vi "Part 1.vi"(11 "Input":string="^^<<v<<v><v^^<><>^^<v<v^>>^^^><^>v^>v><><><<vv^^<^>^^<v^>v>v^v>>>^<>v<^<v^><^>>>>><<v>>^>>^>v^>><<^>v>v<>^v^v^vvv><>^^>v><v<><>^><^^<vv^v<v>^v>>^v^>v><>v^<vv>^><<v^>vv^<<>v>>><<<>>^<vv<^<>^^vv>>>^><<<<vv^v^>>><><^>v<>^>v<v^v<^vv><^v^><<<<>^<>v>^v>v<v<v<<>v<^<<<v>>>>>^^v>vv^^<>^<>^^^^<^^^v<v^^>v<^^v^^>v>^v^^^^>><<v<>v<>^v^<v<>><>^^><<^^<^^>vv<>v^<^v<vv<<<>^>^^>^<>v^^vv<>>v><<<>vvv<>v<>><^<^v<>^vv>^^v<v<v><^<>>vv<^>>^>>vv^v<vv^vv<^<<>>^v^<>^>>>>vv>^^>v>vv>v><^vv^<<v>^<<^^<v<v>vv<v^^<>^^v>^>>v><^<<vv<<v^vv^^^v>>v<<v^><vv^><vv<^vv<<vv^v<<^v<^^v>><<v^>>^^<>v>><<v<>>^^<v>>^^>>vvv^><<<<<^<^vv<^<><v<<>^^^<<<^>^^^<v<<vv>vv<>^<>v<^v>^<<<v<v<v>>^v<>>v<<^<<v<<>^<<<><><>^>>>>^>v^v<<v<v<<>>vv<^vvv^^^^<vv>vv>^v^^v^<v^v><^vv<^vv>v<^>vv<>>^>^><vv<><^>v>^v>vvv<>^>^v<><>vv>><^v^<><><v>>v^v^><^<^>vv>v<^>vvv>v<<<<<^<v<<vv<^^^<<>>^v<vv<^<>v>^<v<>><><>^<<v>v^>^<vv>><><>>^>^>><^<v>^^>^^>^^v^^<^v^^>v^^>>><<><v<v<<v^vv<><><>^<v>^<<^^v^>v>><>^^^><^vvv<^^^^^v><<><v<^^v><><>>^>vv<vvvv<<>>><v<^^^^v<<^><v>^vv<v^^v^vv<^^>^^<v>><<v^>v<^^>^<^<v<^^v>^<<v>^>>>^v<>v<^^^>vvv^v<<^><>>><vvv^<^^^<^>>v>>><v>^^vvv^vvv<^^^^v^v^<vv^<v>^<<^>v^v^<<><>><^v><v<><<>><<<>^v>v<>^<v^v>^vv>>^<>v^^<<v><^v>>v<>>^v^^>><^>v^<^v^^>><>v^>^v^v<<<v^<v^^v<^>v<><>vv>>>>^>v<>v<<<>^^>vv^v<><v^<>^<<<<>>^^>^v<v^v<<><>^v<>>^v^<<^<^>>>^vv<><v<^^<>v^>>v<^^v<v>>>^>><<><<<>><vv<v>>^v>><^<v><vv>^vv<v<>>><>v^><>vv<^^v^^^v<>><^vvv<<^<>v>>>v>><v><>>><>><v^><v^v<v>^v>v<v>>^^<^>^>v><>vv>^v><<>>>>>>>^<<^vv^^vvvv<^^><<<v<<>vvv<>^><<v<v^v^<<v>v<>>^<vv^<v<v>^<<^^vv>v>^<vv<<>v<v^<>v>>^v^^vvvv>^^>>v^v^^><<^>v>>^^>^<^^<>v<v>vv^vv>v<v>>^v<><^vv^<vv<v^^^v<^v^>>^v>>>^^<^<^>^v^>^>>>^v>^>^^^>>^<>v^^<>^v<<^^>^^<vv<>v<^v^>><^v^>^<>>^vv^vv^>v^<vvvvvv^>><^^<^v<^<v^<<^^<<v^<^>><>v><^v^v^^^v>v^<>^<<v<^^vvv<v>^^>^v^^<><vv^v^>v^<<>>vv<>>>>v>v<>^>>>v<>^^><v<v^^^<>^<^><>^><<v>><>^<<>>><<^<vvv<^><v>>^vv^v>><v<>vv^<<^^<<><v><<^<v<vv<<^v^vv>v^>>>v<<<<v<<>v>^vv<^v><v<v>v<^>^^vv>v><v>><<v<<v^v>>><>^<>><><<^<<^v^v<<v>v>v<v<^^>vv<^v^^^<v^<<<v<>v^><^v>^<^<v>>^<<<v>>v^<><>>^v<>vvv<vvvvv<^^><^>><^^>^>^v^vv<^><<^v>><^^v>^v<>^>vvvv><^>^<<v^^vv<v^^<><>v>^>>^<^<<<^v^^^>^>>^>><><<^>v^^<v>>v<<<<vvv<vvvv^<^<v^^<>^>vvv^<vv^v^v>^<<><v><^v^v^^^>^^>^vv<>v>>v^>vv^vv>v<^v^^>>^v^v<>>^^><<v<<>><>>>^>^<>^^v^^><^<>><<^<vv^^^^^>>vv^<v^<^>>>>v<<><<^>vv>vvv>^<><>>>>vv><<v^v<^^^<<^^^vv^<v<><><<<<>><<v^<>v>v^><>v^v^^><>v>v>^^v<^v<>>^^^^^<v>><v^>^^<v>><v^^>v<^<^>>>^><^^>><<>>^><>^^^>v^^^>^^v^<>^^><^>>><><^>>v<v^>v<^><v<v^<>v<^v>v^<^vv^^><<<><><^v^<v<^^>v>v^>>^^vv^<v>^v>^<^v<>^>^><^<v>^v><^<^<>v^^>^><>>><<v><<><>v<<^v^^<^><>^<><><v>v<^^<v<v>>^^<<>>^<v>><^><^<^>^^v<>v>>><><<>^>v><><<<<v^^^^v<>>^^^v>><<^v>^>>><vv^>>^vv<^<>>^<^^<^v>v<v<<<<<>^<<^<<<<<^<^>>^><<>><>v^v>^<^>v^<><vvv^>^v^v^v><^<v<>vv<<^<>^^^<>^v>^<v^^<v^v>v<>>^>v<<>v<>v^v>v<<<>>v>vv>>v<<>v<>v<^>^>^<v>>v>^>^^^<vv>v<<>>><v>^vvv^^>^^<^vv^^^^>v>^v^>v^^v^>>^v>^vv>^^v^<<<<>^<><^<^<<^^>v^^^v<>>vvv<v>>vv><v<v>^<^v>>^v<vv^<<v<vv><^^v^v>v<>^v<<<^^v^^^<^v>v^v^v>><vvv<<>v<>^v>vv^v>vv<<^v<v>^v>v>><^v<v<>v>>>><<<><vv><>^v^<^vvv>v<>><^v>^>><v>vv<><><>v><>>><^>vv>>^<>v^>>^><<<^><<>^v^>>><><>vv>^<>^>^v^^><^>>><<>v^<^vv>^<^vv>><v<>vv<v><><<^><>v<^^<^>vv^^^^vv<<v><>vv<><v>v<>>>>^><v><>^<><>v<>><<>^^vvv>^^^<><>>vvv^v>><>vv<vv>^^^v^<<>^^v<><<^^v<>^^>^<^^v>>v^v^^>>v>>>^<<^<>^>^^v>>>><vv<<>^v<<vv><<^^vv><^>vv<>>v<v>v^>v>>v^<vv<<<v><v^>vvv^^>vv^<<v>v^>>v^<>>><><<^^<^v>^>>>v>v>^v<>vv><vv<vvv<<v>v>^v<<<>><<><><>v^>>>v^>v^>>vv^^<v>^<>>><^>v^<>^^><v>v<><<<><v^v<<<v<v^>v^v>^>v<^<>v>v^^>>v>vv^v<>>^^^^<>v^>>>>>>>><v<^<<vvv<^v^>^v<^<<>>><<<^<<^>^>v^<>^<<<>v>><^vv^>^>^>>>^<vv><v^^^<v^<v<><v^vvv<>v<vvv^vv<<<v^<^<^vvvv^<<vv<^v><<>^>^<v^v^<^>v^><>>v^>v^>^>>v<>vv^v<<>^^>>vv<>vv>>^v<^vv>^v>v<v^vvv^<<^><>v^<><vv><>v^^><<<><>^>^v^<>><vv<^>v^v>v<>><v<<^>^<vv<^v>^<<v><^<^^vv^<>><v^>^vv^<>>^^^^v>v><^^^v^<<<>^<^<<>><>>v<<^v^>><><v^>>^vv^v>vv>>>>>>^^<<>v^>v^v>^^>>><vv^^^v>^v>>^^^<>><>v^<<<v<vv^^<v^<<<>v>v^^^<vv<>>^v>^v<^<<><>vv>^^^<^^vv<v<<vv>^^>vv>v<<^>^vv><^><v>^^^^v<<vv>v^<<^^>>^^vvvv^v^>vv>>v^<v>vvv<>>^><>>v^^>>^<>>vvvv^>><v^v<^^<^vv>>v<<^<<^><v^^><v^>v^>><<<v>v>v^>^v<v^vv<^^^v<^<vvvvv<<vvv>><>v<v<v<<^v<><<>vv>><v>><^>>^^v>^>><>vv^><<>>vv<<<^<^^>^<<^>>>><v<^v<<<>>v>vv<^>^v><>>v<v^v<>v^vvvv>v^>>v><<^<v>^^v>>vv^^>v>^v>^v^^>^<^vv<v<<^>vv<<^>>^<<^^>>^<^>v^><^vv>^^v><v^>>><>v^v>^v<^><<<>vv><v>v<><>>v^<>^^>^<>^<<^>>vv^><^<v<^^vvv>>v^>>v^>v>vv><>>v<^>><<<v<<vv><v<v<v>v<v>vv^vvv^vv^>^>v><vv<v^^<>>>>vv^>^<>v<^>^<^v>vv<^<<>>^<^<vv><^^<>^<<v^v^>v<<><v>v>><^v<<^vvv>v>v<<^^<^^>v<vv<v<v^v>^^^>^>vv<v<<^^v^<v<^>^^^vv>v<>>>vv>><><^><><<<vvv<<^^v^<v^<<^>>vv>vv^v^>>><v><<v^v>>v>>vv>^^vvv^>^^>^>^>^v<<^vv^>vvv^^vv><^>^v^>^><>v<^^vv<v><v^<><^<>><v>^^v^v>v^vv<>><^v>^<^v>^<>^v>>>><<vv^^^vv^>>><vv^v>>v><^v^vv><<^v<<>^^<v><^v>vvv<><^^><<^v><>^<^v<^^<^vvvv^^>>>>vv>v>>>v<v^><<<<v>>v^><v>>vv^v<vv<>vv<>vvv>>>><>>><>^v<v^v><vvv<<v^^v^v<>>><>>^vv<<v<><<vv<v^>^^vv><^v^v<v^vvv^v>v^^^vv>^><^vvv<<>^vvv^<v<v^v>>>>^<<<><<<<<^v<^^>>>>^>^<v^^^v<vvv<vv^<>v<<<^<^>>v^<v><<><<^^vvv^>v<>>^^>v>^v>>v<v><v>>>>^<^<^>v^v<vv<>^>><>^<<^vvv^^<>^<vvv<>v^>^^<<^>^vv><vvv>>v^v^>v><v>^<^^<>^>^>>>^^vvv^<<>v^<<>><>v<^<^>v^>^vv><v<^<<<^v>^>>^<^v^<<<<^v^><v^v>v^><<v<><<v^<<^<<v<<v><v><><^^^^>v>^^<v>>v<vvv<<<>><>>^><<><^<>>^^>vv<^><^v^><vvv>>>vvv<<vv^<^^^<^>^<>>^>>^v^<^^v>^<v<<>^^v<^vv^><vvv>>^v><<^<v^<><><>>^>vv<<>^^^v^^<v<>><>>vv>v^>vvv^^v<vv<^<^>>^>>^>>v^<<<v^>v^<^v^vv^><^<^v<<v<<>v>^v^<<<v^vv<v<<>^^<v>>>^<v<^>^^v<v>>>><vv<^^<<>><<v<v>^^v^>>^^>>^v^<^v>v^v^v^v^>v^vv<><>^^<>^><^^^<<<^<v>v<<>^<^^^^^v^<^<<^^>^vv<>v^>><>>^>v>v<>^>v<v^>>><>^<><v>>>^>^>>v^><v<>v><^vv^>v<<v>v<><<vv<<v>^><^<v^>v<<v^v<<><v><>v<v><>^^<v<>><<>v>vv<<v>^v<v>vv><><>vv^<<>^>^<^>>>^v>v<^v^^^vv<>>>^<<^>>><<^^v^>v^<^v>vvv>v^^vv>^^>>v<>^<<>^<><^^v^>><>^>v>>^^^<<^^v<>^^>^<>^>><^>^vvv><^>^<^>^>>vv<^>>^v>>^<>>^^>>>v^<v>>v<<v<^>>v^^vv>v><^v^^><vv^v<^>v<<>v^^<><>^>vvv><^^^>^v^>v>>^vvv<^vv>^^>^>>v<>><<^v<<v^>^><>vv^<<^^vv><v>>^<^><^<v>^v<v>^<<>^v^^>v^>>^^^<^vv>v^>>>vv<<>v>>>^>v^^<v^v^^v^>>v<v<<v>^<<>>vv<<^v>v<<vv<<^<^v<^<><^^>v>>v>v^>><vv<^v<^>^>>v>^><<^<<>^v<v>>><^^<^<<<v^^>^>vv<<>^<>^<v^<<^v>vv>^^^v<^v><v<<<<<vv>vv>^^^^>v>v><<^<<<^vv><^<<<><v>><v^v>v<<v^^<v^>v>^v^v^<^<^vv>vvv<^^v<>v<<<<>v<v^<vvv^^^<<^<^<<>^<<><<<>v<^>^^v<^^v^>vv>vvv>v><v^^<<>>^><^>>v<<vv>v<<^^^v<<^v^^><><<<><<>v>^<<>v<<<^v>><v^v<^v<v^vv>v>><<^<><^v^^v<v>^>^>vvvv<<><<>>^<vv>^^><v<>v>v<v^^>^><>>><^><<><<<^<>v^><vv^^^^>>^v^>v^<>>v>^^><^<^v^<v^>>v>^vvv<>>v<v^v><>^vvvv<v^<<v^<<^^vv>><<<<<<v><<<v<v^v^^<v^^<>v<<<<^v<<><<v^<^><v<vv<v^v^<v^^vv<v^v<<<>^<<>vv<v<^>^<<><vv<<vv<v<^<^<>><^^<<>>>vv>>>>>>^v<v<>>v^v^^<v^<<<<>><<^v^^^<>^<vv>>>><>v^v^vvv^>>v>><v^v<<<^v>>^^<<^^vv><<<^^^<<<v><^^>>>>vvv^v<^>^^>v<^<><vv<v<>v>>>^vv<<^<v>^v^>^>^v>v>v^v^>v<<v>><>><v^^<<^>>>><<^v^<>^v<vv><>vvv^>v>v<v<v^>^<><><>^>>><v<<<v^vv><>^>^^<<v^>>v^^>^<v>><>><>v^v^^v>>>>vv>>^v<<^v^<>^>v^^>^^<<vvvvvvv>^<v^<<^<<>><<<^^^v^^^^v<^<>v<^^<>vv^^v^<>^<<^>>v>v<<<^^^^vvv^<^<><>v<<v^<^<>>><<><<<v<v<v><vv>^^<vv<<vv<<<v<^>^^vv<v<>><<>>>^v<<>^>>>v^>v>^^<>^<vv<><^>v>^>>>><>^^>v^^v>^vv^^v^><<<>>v<>v<vv<vv^v^v<^v^<^^><<<><vv^^>^<^<<>v>>>>^<<v>v<v>vv<^><^<v><<^>v>>v><<v<<^v^<>>^>>>^v^v>v^^vv^>^<^^>>^><^vv^^vv^<>>^^^^<^^><><v<>>^>>^><vv^>^vvv<^<<v^^<<<>^><>>>^^<><v<v<><<v^^^^^<^<^<<>><<>>>>^<<>>>^<^v^>><<^>>>^<<v>^>><>^<v>^<><v>^v^^vv<><^>vv^^v^<^^^v^vvv^>><>>v<<vv<>>^<^vvv<<^^><vvv^^<v<>vv^^<<>><v>><^^vvv<<<^>^<><^>vv^><^<<>vv<<v>>vv>v>v^<vv><vv><<>^^^^v^^^^<v>^<<^><><^^v^>v>^>><^><<>v^<v>>>^vvv>>^<^<>^^v^vv^^v><<vv^<>>>v<<<>v>^<>v<<>v^>^<<><<><v<v<v<>v^>v<><^^>^<^v^^><^>vv>^>vv<v<^v>vv>^^><<>vv^>^v<<^<<^<<>v<v<^<v>v>>^><v^^v^v>>>><v^v^<<<vv<<^^<>>v^v<^v>v>^^^v<v><v^^^vv<>v^v<^<>v><><v^<>>vv>v><>v>^v<><<<<<<v<>>v^vv<<<<v<<v><^<>^>><>^^vv>^<^<<>vv>>vv<vvv>><><v<>><^<v>^><^<<v>><v><v>^<v>><>v^^^^v<v^^v<>^^vv<>v<>v>^vv^><v^<<^<>^<>^^^>v^>>>v><<^>>v<^v<>^^<v<><v^v<v>v<><v<vv><<>v<^<^>v<>v^>v>^^<<<^^vv^<><<<>>v>^^<>v>>>><v<v<^^^v<v<v^><<>v^v<>v>><<<<v^<><^<<^>^<vvv<v^^v>>v^vv^><^v^^<>^^><<v^>>vv>^<v^vv<^^v<>>vvv<^v^>>^<v<v>>^>^^<<^>^>^v><>>^<^^v>^>>^^<><>>>^^>^^vvv>v<^^<>v^v^^<v<<^<v^v^<<>v^v<v<<v<>>><<^^^>>v>^vv>^>^^v<>^^<>v^^<><v<v<vvv^<vv<<>v^><<><v<>vv<<^vvvv><<<v>v>v^>v^<>v^>^<v<vvv^>^<>^>^^v<>><<<><v<^^>^v<v>^^v^v<<<^v^<>^<>v>^^>v<v<v>v>^^<<<><<^>v<v<^vv^v><^^<<vv>^<<v><>^>>>>><v^v<<<^>^v^v<<v<>vvv<<>v>v>>^v^v^>><<<<>v^<v<><<>>>^>>^>><<v>") -> (3 "Output":i64)   [LabVIEW 2021]
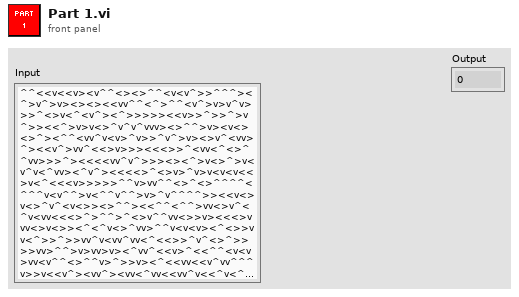
[diagram p1: front panel]
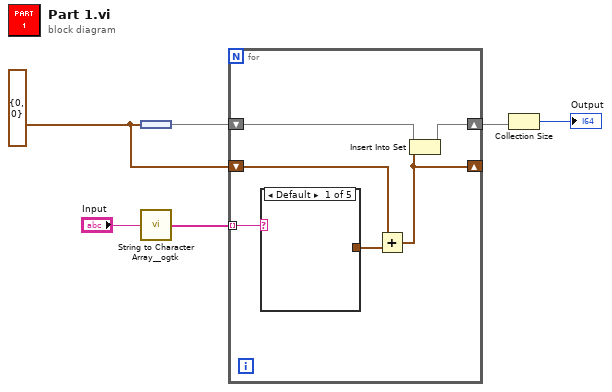
[diagram p0: block diagram]
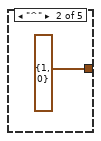
[diagram p2: hidden frame]
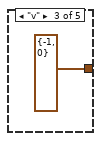
[diagram p3: hidden frame]
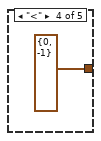
[diagram p4: hidden frame]
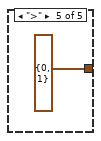
[diagram p5: hidden frame]
diagram:
  w3 = cluster{"X":i32, "Y":i32} {"X"=0, "Y"=0}
  n1 = node(w3) -> (w4:set{cluster{"X":i32, "Y":i32}})
  n2 = call <userlib>:"String to Character Array__ogtk.vi"("Input String"="Input") -> ("Character Array"=w5:string[])
  n3 = for {
    tunnel: w5 -> [w12] mode=indexing
    shift-right: [w8] -> w2
    shift-left: w4 -> [w9]
    shift-right: [w7] -> _
    shift-left: w3 -> [w10]
    n4 = case shown="Default" w12 {
      tunnel: [_ cluster{"X":i32, "Y":i32} {"X"=1, "Y"=0} cluster{"X":i32, "Y":i32} {"X"=-1, "Y"=0} cluster{"X":i32, "Y":i32} {"X"=0, "Y"=-1} cluster{"X":i32, "Y":i32} {"X"=0, "Y"=1}] -> w11
      frame Default {
      }
      frame "^" {
      }
      frame "v" {
      }
      frame "<" {
      }
      frame ">" {
      }
    }
    n5 = Add(x=w10, y=w11) -> (x+y=w7:cluster{"X":i32, "Y":i32})
    n6 = Insert Into Set(10:w7, 11:w9) -> (3:w8:set{cluster{"X":i32, "Y":i32}})  [unwired: 1 out]
  }
  n7 = Collection Size(1:w2) -> (0:→"Output":i32)
